vi "PWM Command Test.vi"(8 "error in (no error)":errorcluster, 10 "VISA resource name":refnum<visa-resource-name>, 11 "Leg":i32 min=0 max=6) -> (0 "error out":errorcluster)   [LabVIEW 2022 SP3]
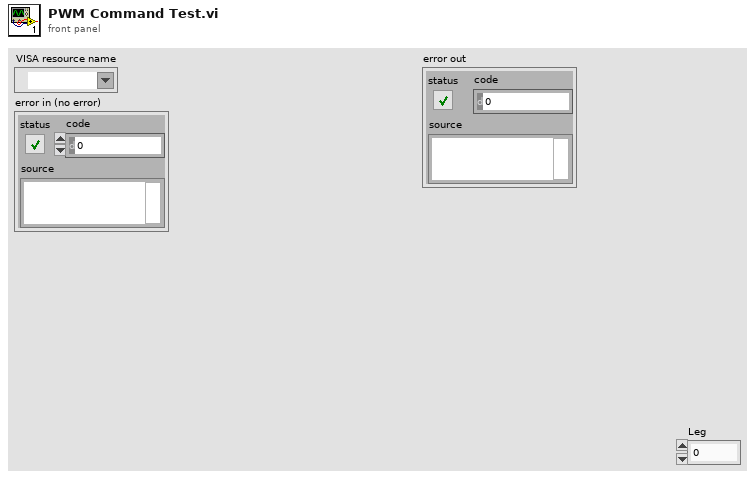
[diagram p1: front panel]
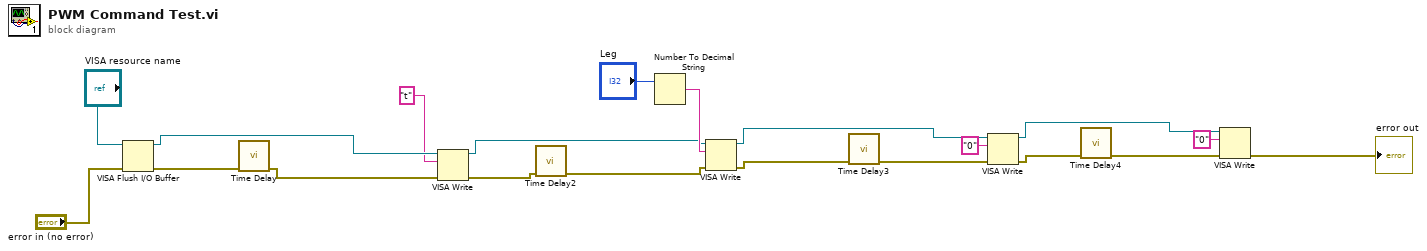
[diagram p0: block diagram]
diagram:
  n1 = VISA Flush I/O Buffer(VISA resource name="VISA resource name", error in (no error)="error in (no error)") -> (VISA resource name out=w17:refnum<visa-resource-name>, error out=w18:errorcluster)  [unwired: 1 in]
  n2 = call "Time Delay"("error in (no error)"=w18) -> ("error out"=w16:errorcluster)  [unwired: 10 in]
  n3 = VISA Write(VISA resource name=w17, write buffer="t", error in (no error)=w16) -> (VISA resource name out=w10:refnum<visa-resource-name>, error out=w14:errorcluster)  [unwired: 1 out]
  n4 = call "Time Delay2"("error in (no error)"=w14) -> ("error out"=w11:errorcluster)  [unwired: 10 in]
  n5 = Number To Decimal String(number="Leg") -> (decimal integer string=w12:string)  [unwired: 1 in]
  n6 = VISA Write(VISA resource name=w10, write buffer=w12, error in (no error)=w11) -> (VISA resource name out=w8:refnum<visa-resource-name>, error out=w9:errorcluster)  [unwired: 1 out]
  n7 = call "Time Delay3"("error in (no error)"=w9) -> ("error out"=w6:errorcluster)  [unwired: 10 in]
  n8 = VISA Write(VISA resource name=w8, write buffer="0", error in (no error)=w6) -> (VISA resource name out=w2:refnum<visa-resource-name>, error out=w3:errorcluster)  [unwired: 1 out]
  n9 = call "Time Delay4"("error in (no error)"=w3) -> ("error out"=w4:errorcluster)  [unwired: 10 in]
  n10 = VISA Write(VISA resource name=w2, write buffer="0", error in (no error)=w4) -> (error out=→"error out":errorcluster)  [unwired: 2 out]
